vi "Run.vi"(8 "error in (no error)":errorcluster caption="entrée d'erreur (pas d'erreur)", 10 "patches":cluster{"Array":i32[][]}[](array[cluster]), 11 "Reconstruct_from_patches_2d.lvclass":refnum<class "Reconstruct_from_patches_2d.lvclass">) -> (0 "error out":errorcluster caption="sortie d'erreur", 2 "Data":T1, 3 "Reconstruct_from_patches_2d.lvclass":refnum<class "Reconstruct_from_patches_2d.lvclass">)   [LabVIEW 2020, in "Reconstruct_from_patches_2d.lvclass"]
doc: "Returns : \n\n- image : ndarray of shape image_size\nThe reconstructed image."
uses:
  Reconstruct_from_patches_2d.lvclass
  Reconstruct_from_patches_2d.lvclass/Reconstruct_from_patches_2d.ctl
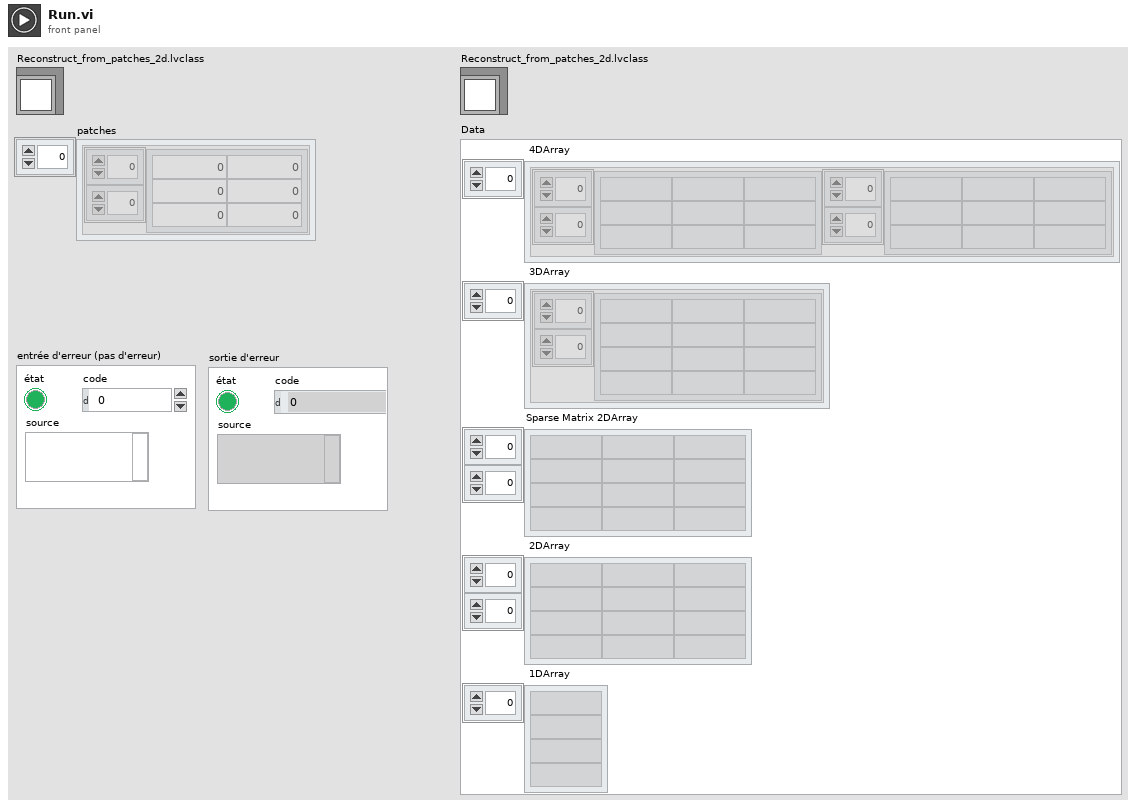
[diagram p1: front panel]
types:
  T1 = cluster{" 4DArray":cluster{"1":string[][], "2":string[][]}[], " 3DArray":cluster{"Tableau":string[][]}[], "Sparse Matrix 2DArray":string[][], " 2DArray":string[][], " 1DArray":string[]}
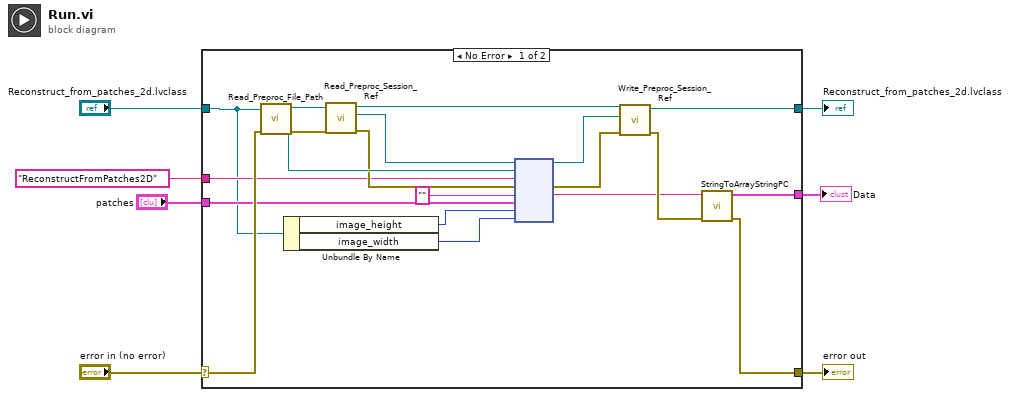
[diagram p0: block diagram]
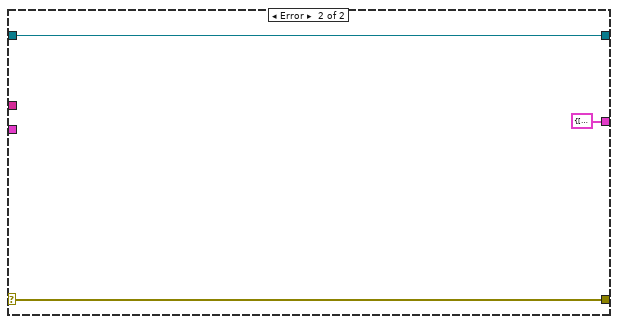
[diagram p2: hidden frame]
diagram:
  n1 = case shown="No Error" "error in (no error)" {
    selector: "error in (no error)" -> [w18 w30]
    tunnel: [w11 w30] -> w6
    tunnel: [w15 w29] -> w4
    tunnel: "Reconstruct_from_patches_2d.lvclass" -> [w10 w29]
    tunnel: "ReconstructFromPatches2D" ("Fonction") -> [w17 _]
    tunnel: "patches" -> [w16 _]
    tunnel: [w12 T1 {" 4DArray"=[], " 3DArray"=[], "Sparse Matrix 2DArray"=[], " 2DArray"=[], " 1DArray"=[]} ("Data")] -> w1
    frame No Error {
      n2 = call-dynamic "Read_Preproc_File_Path.vi"("error in (no error)"=w18, "Python in"=w10) -> ("error out"=w26:errorcluster, "File_Path"=w25:path, "Python out"=w27:refnum<class "Reconstruct_from_patches_2d.lvclass">)  [unwired: 7 in]
      n3 = Unbundle By Name(w10) -> ("image_height"=w9:i32, "image_width"=w8:i32)
      n4 = call-dynamic "Read_Preproc_Session_Ref.vi"("error in (no error)"=w26, "Python in"=w27) -> ("error out"=w23:errorcluster, "Session_ref"=w24:refnum<k35>, "Python out"=w22:refnum<class "Reconstruct_from_patches_2d.lvclass">)  [unwired: 7 in]
      n5 = node(w24, w25, w17, w23, "", w16, w9, w8) -> (w20:refnum<k35>, w21:errorcluster, w13:string)  [unwired: 3 in, 2 out]
      n6 = call-dynamic "Write_Preproc_Session_Ref.vi"("error in (no error)"=w21, "Session_ref"=w20, "Python in"=w22) -> ("error out"=w14:errorcluster, "Python out"=w15:refnum<class "Reconstruct_from_patches_2d.lvclass">)  [unwired: 7 in]
      n7 = call "StringToArrayStringPC.vi"("sortie d'erreur"=w14, "Return value"=w13) -> ("sortie d'erreur"=w11:errorcluster, "Data"=w12:T1)  [unwired: 8 in]
    }
    frame Error {
    }
  }
  "error out" <- w6
  "Reconstruct_from_patches_2d.lvclass" <- w4
  "Data" <- w1
